vi "InitOpen.vi"() -> (0 "error out":errorcluster, 2 "OscilloscopeCluster":T1, 3 "hDevice":u32)   [LabVIEW 2018]
uses:
  LibTiePie.lvlib
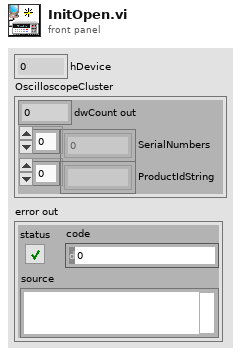
[diagram p1: front panel]
types:
  T1 = cluster{"dwCount out":u32, "SerialNumbers":u32[], "ProductIdString":string[]}
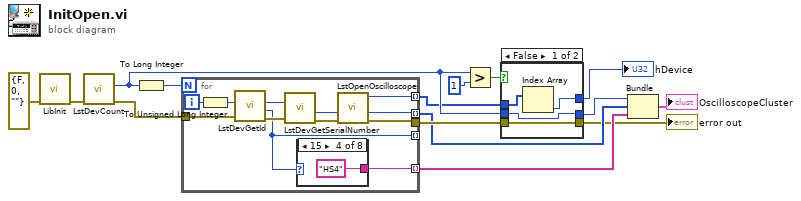
[diagram p0: block diagram]
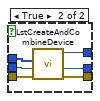
[diagram p2: hidden frame]
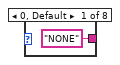
[diagram p3: hidden frame]
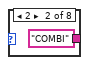
[diagram p4: hidden frame]
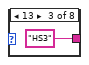
[diagram p5: hidden frame]
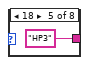
[diagram p6: hidden frame]
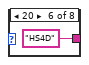
[diagram p7: hidden frame]
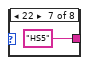
[diagram p8: hidden frame]
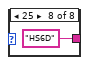
[diagram p9: hidden frame]
diagram:
  n1 = call "LibInit.vi"("error in (no error)"=errorcluster {"status"=FALSE, "code"=0, "source"=""} ("error in")) -> ("error out"=w14:errorcluster)  [unwired: 10 in]
  n2 = call "LstDevCount.vi"("error in (no error)"=w14) -> ("error out"=w12:errorcluster, "Count"=w8:u32)  [unwired: 9 in]
  n3 = To Long Integer(number=w8) -> (32bit integer=w13:i32)
  n4 = for {
    N: w13 -> [_]
    tunnel: w12 -> [w27]
    tunnel: [w17] -> _ mode=indexing
    tunnel: [w20] -> w7 mode=indexing
    tunnel: [w19] -> w6 mode=indexing
    tunnel: [w18] -> w9
    tunnel: [w16] -> w5 mode=indexing
    i -> [w25]
    n5 = To Unsigned Long Integer(number=w25) -> (unsigned 32bit integer=w26:u32)
    n6 = call "LstDevGetId.vi"("error in (no error)"=w27, "dwId in"=w26) -> ("error out"=w24:errorcluster, "dwProductId"=w17:u32, "dwId out"=w23:u32)  [unwired: 6 in]
    n7 = call "LstDevGetSerialNumber.vi"("error in (no error)"=w24, "dwId in"=w23) -> ("error out"=w21:errorcluster, "Serial No."=w22:u32)  [unwired: 7 in, 1 out]
    n8 = case shown="15" w17 {
      tunnel: ["NONE" "COMBI" "HS3" "HS4" "HP3" "HS4D" "HS5" "HS6D"] -> w16
      frame 0, Default {
      }
      frame 2 {
      }
      frame 13 {
      }
      frame 15 {
      }
      frame 18 {
      }
      frame 20 {
      }
      frame 22 {
      }
      frame 25 {
      }
    }
    n9 = call "LstOpenOscilloscope.vi"("error in (no error)"=w21, "dwSerialNumber in"=w22) -> ("error out"=w18:errorcluster, "dwSerialNumber out"=w19:u32, "hDevice"=w20:u32)  [unwired: 7 in]
  }
  n10 = Greater?(x=w8, y=u32 1) -> (0:w10:bool)
  n11 = case shown="False" w10 {
    tunnel: w9 -> [w38 w45]
    tunnel: w8 -> [w36 w44]
    tunnel: w7 -> [w39 w43]
    tunnel: [w38 w42] -> w4
    tunnel: [w37 w41] -> w1
    tunnel: [w36 w40] -> w2
    frame False {
      n12 = Index Array(array=w39) -> (element=w37:u32)  [unwired: 1 in]
    }
    frame True {
      n13 = call "LstCreateAndCombineDevice.vi"("error in (no error)"=w45, "dwCount in"=w44, "pDevicesHandles in"=w43) -> ("error out"=w42:errorcluster, "dwCount out"=w40:u32, "hDevice"=w41:u32)  [unwired: 5 in, 1 out]
    }
  }
  "error out" <- w4
  "hDevice" <- w1
  n14 = Bundle("dwCount out"=w2, w6, w5) -> (→"OscilloscopeCluster":cluster{"dwCount out":u32, u32[], string[]})  [unwired: 1 in]
